vi "XML generator.vi"(8 "error in (no error)":errorcluster, 11 "vi":refnum<vi>) -> (0 "error out":errorcluster, 2 "XML":string, 3 "vi out":refnum<vi>)   [LabVIEW 2021, in "NI Measurement Plug-In SDK.lvlib"]
uses:
  NI Measurement Plug-In SDK.lvlib
  <vilib>/regexp/Match Regular Expression.xnode
panel:
  in  "vi path":path
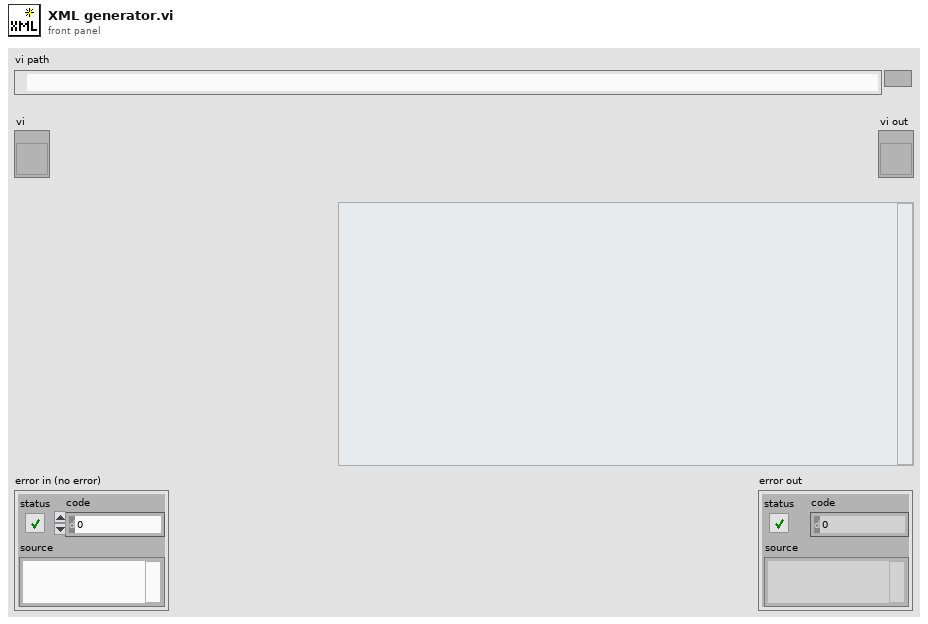
[diagram p1: front panel]
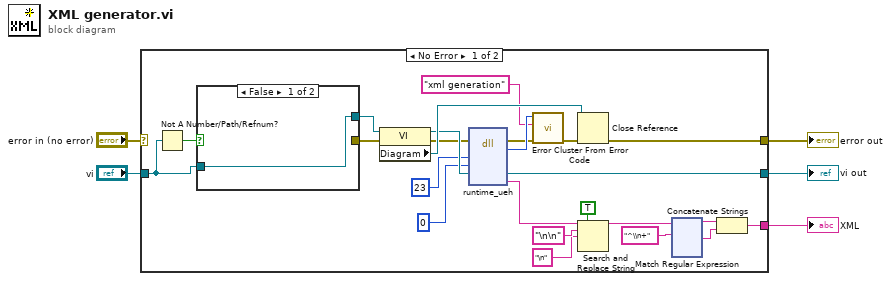
[diagram p0: block diagram]
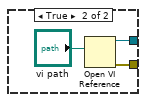
[diagram p2: hidden frame]
diagram:
  n1 = case shown="No Error" "error in (no error)" {
    selector: "error in (no error)" -> [_ w152]
    tunnel: "vi" -> [w20 w151]
    tunnel: [w13 _] -> w3
    tunnel: [w11 w152] -> w2
    tunnel: [w6 w151] -> w1
    frame No Error {
      n2 = Not A Number/Path/Refnum?(number/path/refnum=w20) -> (NaN/Path/Refnum?=w27:bool)
      n3 = case shown="False" w27 {
        tunnel: [w30 w32] -> w28
        tunnel: w20 -> [w30 _]
        tunnel: [_ w31] -> w29
        frame False {
        }
        frame True {
          n4 = Open VI Reference(vi path="vi path") -> (vi reference=w32:refnum<vi>, error out=w31:errorcluster)  [unwired: 5 in]
        }
      }
      n5 = property class="VI"(reference=w28, error in=w29) -> (reference out=w21:refnum<vi>, error out=w12:errorcluster, "Diagram"=w22:refnum<vi>)
      n6 = dll-call lib="LabVIEW" fn="runtime_ueh"(error in=w12, "selector"=23, "flags"=u64 0, "input"=w21) -> (error out=w9:errorcluster, "mgErr"=w10:i32, "input"=w6:refnum<vi>, "output"=w23:string)  [unwired: 5 in, 1 out]
      n7 = call <vilib>:"Error Cluster From Error Code.vi"("error in (no error)"=w9, "error message (\"\")"="xml generation" ("error message (\"\")"), "error code (0)"=w10) -> ("error out"=w8:errorcluster)  [unwired: 6 in]
      n8 = Close Reference(reference=w22, error in (no error)=w8) -> (error out=w11:errorcluster)
      n9 = Search and Replace String(replace all?=TRUE ("replace all? (F)"), input string=w23, search string="\n\n", replace string="\n" ("replace string (\"\")")) -> (result string=w26:string)  [unwired: 4 in, 3 out]
      n10 = xnode "Match Regular Expression"("input string"=w26, "regular expression"="^\\n+") -> ("before match"=w24:string, "after match"=w25:string)  [unwired: 4 in, 3 out]
      n11 = Concatenate Strings(w24, w25) -> (w13:string)
    }
    frame Error {
    }
  }
  "XML" <- w3
  "error out" <- w2
  "vi out" <- w1
